vi "PWM Servo position FPGA.vi"() -> ()   [LabVIEW 2014]
doc: "This VI shows an example of how to implement a closed loop position move using the NI 9505. The position loop is implemented using PID. The output of the loop is used as the command for the current loop, which then sets the PWM duty cycle for the motor. This example assumes that an encoder is connected for position and velocity feedback. This example does not implement advanced motion features such as trajectory generation and splining."
uses:
  <vilib>/LabVIEW Targets/FPGA/cRIO/cRIO-9505/controls.llb/_nicrio_cRIO-9505_DriveStatus.ctl
  <vilib>/Platform/TimedLoop/XDataNode/timing_clust.ctl
  <vilib>/Platform/TimedLoop/XDataNode/nitl_modes.ctl
  <vilib>/Platform/TimedLoop/XDataNode/wakeup.ctl
  <vilib>/LabVIEW Targets/FPGA/cRIO/cRIO-9505/controls.llb/_nicrio_cRIO-9505_DriveDirection.ctl
  <vilib>/rvi/Emulation/niFpgaGetClockAttributes.vi
  <vilib>/rvi/Emulation/niFpgaSctlEmulationGetInTimedLoop.vi
  <vilib>/rvi/Emulation/niFpgaEmulationReportErrorSimple.vi
  <vilib>/rvi/eio/common/nirviEmuTemplateMethod_errors.vi
  <vilib>/rvi/eio/common/nirviEmuTemplatePropertyGet_noerrors.vi
  <vilib>/rvi/Emulation/niFpgaCriticalErrorInLSC.vi
  <vilib>/rvi/Emulation/niFpgaProcessEmulError.vi
  Instance           3 55Saved   Position Control (closed loop) - NI 9505 (FPGA) .vi
  Instance           4 55Saved   Position Control (closed loop) - NI 9505 (FPGA) .vi
  Instance           1 55Saved   Position Control (closed loop) - NI 9505 (FPGA) .vi
  Instance           2 55Saved   Position Control (closed loop) - NI 9505 (FPGA) .vi
  <vilib>/eio/EIOMethodNode/EIOMethodNode.xnode
  <vilib>/eio/EIOPropertyNode/EIOPropertyNode.xnode
  <vilib>/Platform/TimedLoop/XDataNode/XDataNode.xnode
  <vilib>/eio/EIONode/EIONode.xnode
  <vilib>/Platform/TimedLoop/XDataNode/XDNodeRunTimeDep.lvlib
  <vilib>/rvi/eio/common/nirviEmuTemplatePropertyGet_errors.vi
  <vilib>/rvi/eio/common/nirviEmuTemplatePropertySet_errors.vi
  <vilib>/rvi/eio/common/nirviEmuTemplatePropertySet_noerrors.vi
panel:
  out "Vsup Present":bool
  out "Drive Fault":bool
  out "Drive Status":T1=enum."Disabled"
  out "Temp Fault":bool
  in  "Enable\nDrive":bool
  in  "Disable\nDrive":bool
  in  "Reset Position":bool
  in  "Reset Position Value":i32
  out "Encoder Position":i32
  out "ticks/count":u32
  out "Index (Z) Position":i32
  out "counts (no reset)":i32
  in  "Position Loop  Rate (usec)":u16=250
  in  "Position PID Gains":T2={"Kp"=100, "Kd"=1000, "Ki"=0, "ILim"=1000, "Kv"=0, "Vff"=0, "Aff"=0, "Td"=2}
  in  "Position Error Limit":i16=32767
  out "Position Error Read":i16
  out "Position Error Status":bool
  in  "Position Setpoint":i32 caption="Setpoint"
  in  "Current PI Gains":T3={"Proportional Gain"=20, "Integral Gain"=10, "Derivative Gain"=0}
  in  "Current Limit":i16 caption="Setpoint"
  in  "Current Loop\nRate (usec)":u32=50
  in  "Trig AI":bool
  in  "Current Feedback":i16
  out "Current Loop Output":i16
  out "Current Command":i16
  # "VI Execution\nThis VI should be run with \"Position Control (closed loop) - NI 9505 (RT).vi\"."
  # "These parameters control the response of the position loop. Position Setpoint is the desired position to go to. Position Error Limit is the maximum allowed error the setpoint and actual position returned by the encoder loop."
  # "These parameters control the response\nof the current loop. The current limit is the \nmaximum current allowed."
  # "Kp: 3000\nKd: 2000\nKi: 1000\nILim: 1\n\nLoop rate: 50\nLimit: 100"
  # "Use the Reset Position control to reset the quadrature count to the value in Reset Position Value."
  # "These status controls/indicators are used to enable/disable the drive and read fault information."
  # "Drive Status"
  # "Encoder Parameters"
  # "Position Loop Parameters"
  # "Current Loop Parameters"
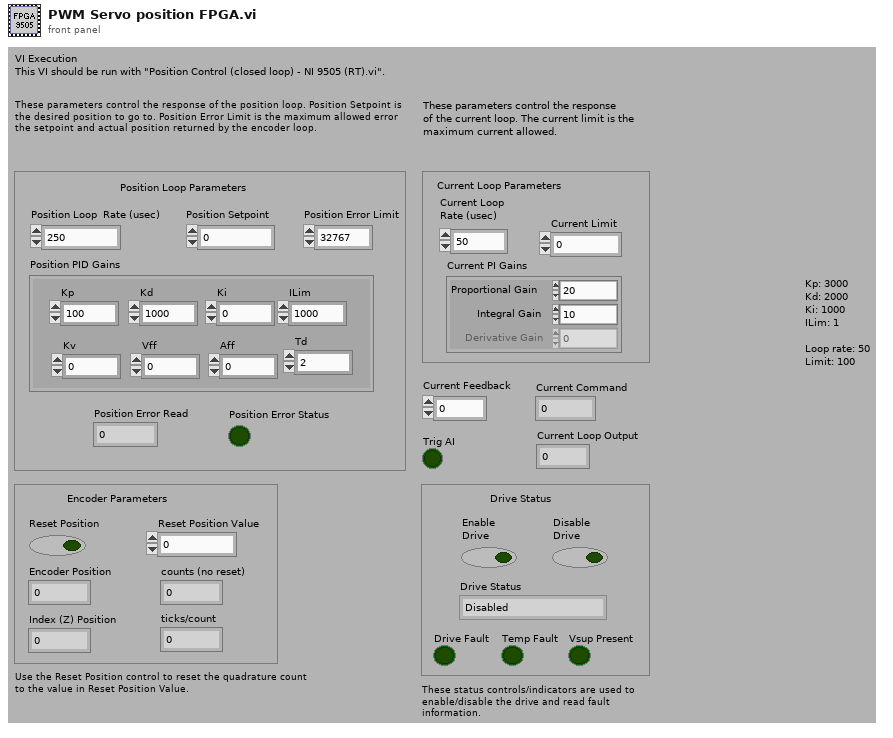
[diagram p1: front panel]
types:
  T1 = typedef "_nicrio_cRIO-9505_DriveStatus.ctl" = enum8{"Enabled", "Disabled", "Disabled by Drive Fault", "Disabled by Temp. Fault", "Disabled by E-Stop", "Unknown"}
  T2 = cluster{"Kp":i16, "Kd":i16, "Ki":i16, "ILim":i16, "Kv":i16, "Vff":i16, "Aff":i16, "Td":i16}
  T3 = cluster{"Proportional Gain":i16, "Integral Gain":i16, "Derivative Gain":i16}
  T4 = typedef "XDNodeRunTimeDep.lvlib/timing_clust.ctl" = cluster{"Expected End [f-1]":u64, "Actual End [f-1]":u64, "Finished Late? [f-1]":bool, "Expected End [i-1]":u64, "Actual End [i-1]":u64, "Finished Late? [i-1]":bool, "Expected Start [i]":u64, "Actual Start [i]":u64, "Expected Start [f]":u64, "Actual Start [f]":u64, "Source Name":string, "Structure Name":string, "Period":i64, "Deadline":i64, "Offset":i64, "Start":i64, "Priority":i32, "Timeout":i32, "Mode":T5, "Wakeup Reason":T6, "Error":errorcluster, "Source Type":string, "Secondary Source Type":string, "Global End Time":u64, "Global Start Time":u64, "Frame Duration":u64, "Iteration Duration":u64, "Assigned CPU":i32, "I/O Scan Engine Mode":u32}
  T5 = typedef "XDNodeRunTimeDep.lvlib/nitl_modes.ctl" = enum32{"No Change", "Process missed periods, maintain original phase", "Discard missed periods, maintain original phase", "Process missed periods, ignore original phase", "Discard missed periods, ignore original phase"}
  T6 = typedef "XDNodeRunTimeDep.lvlib/wakeup.ctl" = enum32{"Normal", "Aborted", "Asynchronous wakeup", "Timing source error", "Timed loop error", "Timeout"}
  T7 = typedef "_nicrio_cRIO-9505_DriveDirection.ctl" = enum8{"Clockwise", "Counterclockwise"}
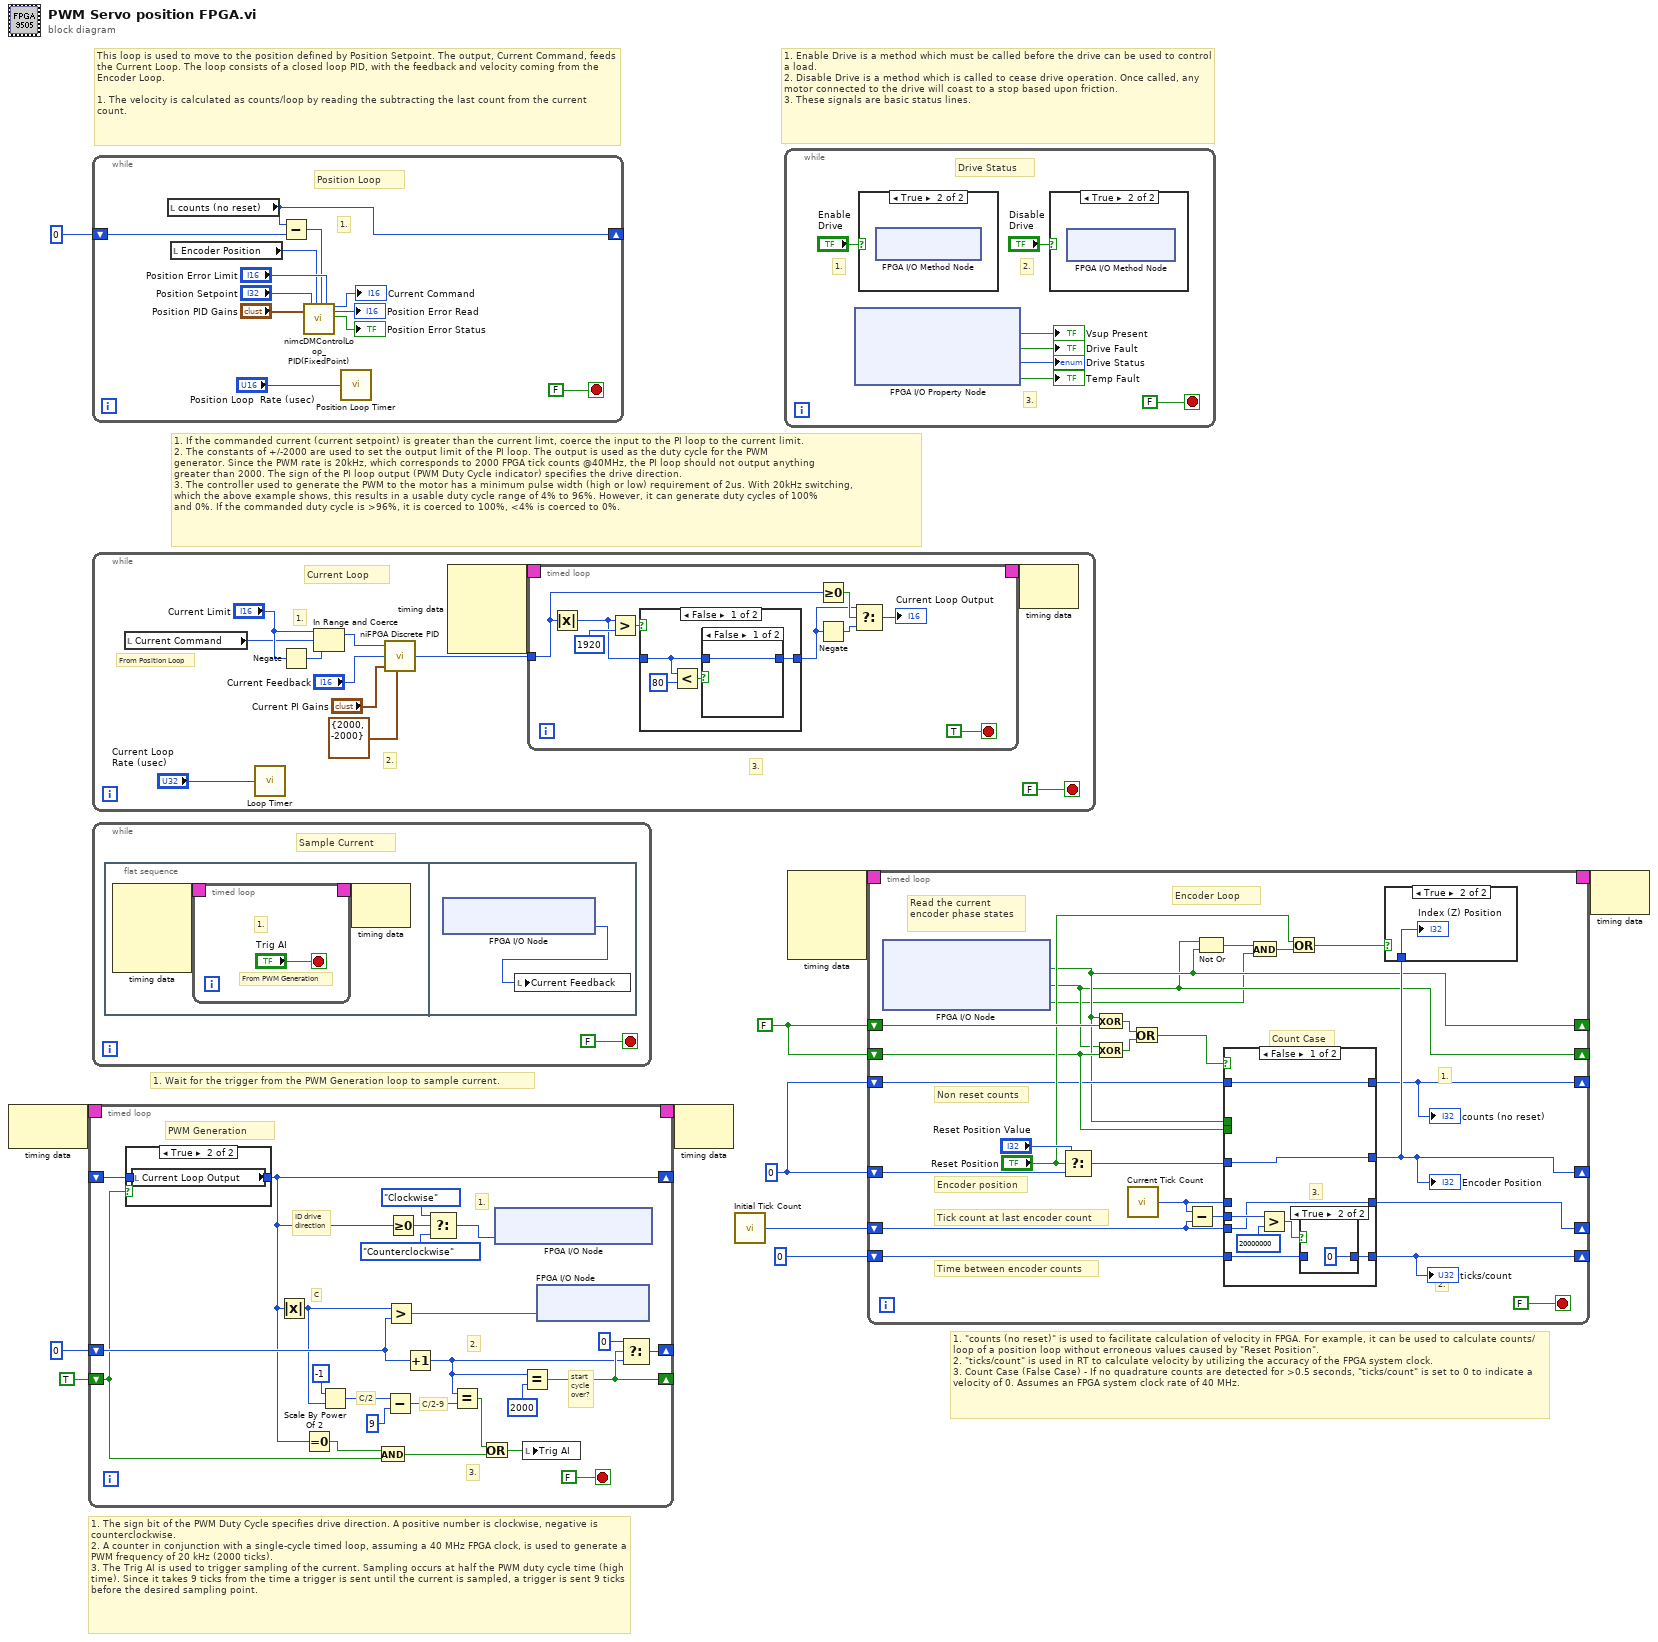
[diagram p0: block diagram]
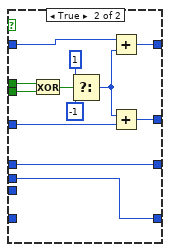
[diagram p4: hidden frame]
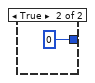
[diagram p6: hidden frame]
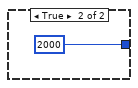
[diagram p7: hidden frame]
diagram:
  w2 = 0 ("Reset Position Value")
  w5 = FALSE ("Encoder Phase A")
  # "1. \"counts (no reset)\" is used to facilitate calculation of velocity in FPGA. For example, it can be used to calculate counts/loop of a position loop without erroneous values caused by \"Reset Position\". \n2. \"ticks/count\" is used in RT to calculate velocity by utilizing the accuracy of the FPGA system clock.\n3. Count Case (False Case) - If no quadrature counts are detected for >0.5 seconds, \"ticks/count\" is set to 0 to indicate a velocity of 0. Assumes an FPGA system clock rate of 40 MHz."
  # "1. Enable Drive is a method which must be called before the drive can be used to control a load.\n2. Disable Drive is a method which is called to cease drive operation. Once called, any motor connected to the drive will coast to a stop based upon friction.\n3. These signals are basic status lines."
  # "This loop is used to move to the position defined by Position Setpoint. The output, Current Command, feeds the Current Loop. The loop consists of a closed loop PID, with the feedback and velocity coming from the Encoder Loop.\n\n1. The velocity is calculated as counts/loop by reading the subtracting the last count from the current count."
  # "1. The sign bit of the PWM Duty Cycle specifies drive direction. A positive number is clockwise, negative is counterclockwise. \n2. A counter in conjunction with a single-cycle timed loop, assuming a 40 MHz FPGA clock, is used to generate a PWM frequency of 20 kHz (2000 ticks).\n3. The Trig AI is used to trigger sampling of the current. Sampling occurs at half the PWM duty cycle time (high time). Since it takes 9 ticks from the time a trigger is sent until the current is sampled, a trigger is sent 9 ticks before the desired sampling point."
  # "1. Wait for the trigger from the PWM Generation loop to sample current."
  # "1. If the commanded current (current setpoint) is greater than the current limt, coerce the input to the PI loop to the current limit.\n2. The constants of +/-2000 are used to set the output limit of the PI loop. The output is used as the duty cycle for the PWM\ngenerator. Since the PWM rate is 20kHz, which corresponds to 2000 FPGA tick counts @40MHz, the PI loop should not output anything\ngreater than 2000. The sign of the PI loop output (PWM Duty Cycle indicator) specifies the drive direction.\n3. The controller used to generate the PWM to the motor has a minimum pulse width (high or low) requirement of 2us. With 20kHz switching,\nwhich the above example shows, this results in a usable duty cycle range of 4% to 96%. However, it can generate duty cycles of 100%\nand 0%. If the commanded duty cycle is >96%, it is coerced to 100%, <4% is coerced to 0%."
  n1 = node-c288() -> (w11:T4)  [unwired: 1 out]
  n2 = timed-loop {
    timing: w11 -> [_]
    timing-out: [_] -> w10
    shift-right: [w32] -> _
    shift-left: i16 0 -> [w35]
    shift-right: [w31] -> _
    shift-left: TRUE -> [w28]
    shift-right: [w16] -> _
    shift-left: _ -> [w30]
    stop <- FALSE stop-if-true
    # "start \ncycle \nover?"
    # "C/2-9"
    # "C/2"
    # "C"
    # "ID drive\ndirection"
    # "3."
    # "2."
    # "1."
    # "PWM Generation"
    n3 = case shown="True" w28 {
      tunnel: [w36 w37] -> w16
      tunnel: w30 -> [w36 _]
      frame False {
      }
      frame True {
        n4 = local read "Current Loop Output"() -> (w37:i16)
      }
    }
    n5 = Absolute Value(x=w16) -> (abs(x)=w14:i16)
    n6 = Equal To 0?(x=w16) -> (x = 0?=w29:bool)
    n7 = Scale By Power Of 2(n=i8 -1, x=w14) -> (x*2^n=w18:i16)
    n8 = And(x=w29, y=w28) -> (x .and. y?=w25:bool)
    n9 = Subtract(x=w18, y=i8 9) -> (x-y=w17:i16)
    n10 = Greater?(x=w14, y=w35) -> (0:w12:bool)
    n11 = Greater Or Equal To 0?(x=w16) -> (x >= 0?=w24:bool)
    n12 = Increment(x=w35) -> (x+1=w27:i16)
    n13 = Select(t=_nicrio_cRIO-9505_DriveDirection."Clockwise" ("Drive Direction"), s=w24, f=_nicrio_cRIO-9505_DriveDirection."Counterclockwise" ("Drive Direction")) -> (s? t:f=w13:T7)
    n14 = Equal?(x=w27, y=w17) -> (x = y?=w26:bool)
    n15 = Or(x=w26, y=w25) -> (x .or. y?=w20:bool)
    n16 = xnode "FPGA I/O Node"("Mod7/Drive Direction"=w13) -> ()  [unwired: 1 in, 1 out]
    n17 = Equal?(x=w27, y=i16 2000) -> (x = y?=w31:bool)
    n18 = local write "Trig AI"(w20) -> ()
    n19 = xnode "FPGA I/O Node"("Mod7/Motor"=w12) -> ()  [unwired: 1 in, 1 out]
    n20 = Select(t=i16 0, s=w31, f=w27) -> (s? t:f=w32:i16)
  }
  n21 = while "Position Control Loop" {
    shift-right: [w43] -> _
    shift-left: 0 ("Encoder Position") -> [w45]
    stop <- FALSE stop-if-true
    # "1."
    # "Position Loop"
    n22 = local read "counts (no reset)"() -> (w43:i32)
    n23 = local read "Encoder Position"() -> (w40:i32)
    n24 = Subtract(x=w43, y=w45) -> (x-y=w44:i32)
    n25 = call "nimcDMControlLoop_PID(FixedPoint).vi"("PID Gains"="Position PID Gains", "Setpoint"="Position Setpoint", "Position Feedback"=w40, "Velocity Feedback"=w44, "Position Error Limit"="Position Error Limit") -> ("Output"=→"Current Command":i16, "Position Error Read"=→"Position Error Read":i16, "Position Error Status"=→"Position Error Status":bool)  [unwired: 2 in, 10 out]
    n26 = call "Position Loop Timer"("Count(uSec)"="Position Loop  Rate (usec)") -> ()  [unwired: 1 out]
  }
  n27 = while {
    stop <- FALSE stop-if-true
    # "From Position Loop"
    # "3."
    # "2."
    # "1."
    # "Current Loop"
    n28 = local read "Current Command"() -> (w52:i16)
    n29 = call "Loop Timer"("Count(uSec)"="Current Loop\nRate (usec)") -> ()  [unwired: 1 out]
    n30 = Negate(x="Current Limit") -> (-x=w56:i16)
    n31 = In Range and Coerce(upper limit="Current Limit", x=w52, lower limit=w56) -> (coerced(x)=w54:i16)  [unwired: 1 out]
    n32 = call <vilib>:"niFPGA Discrete PID.vi"("setpoint"=w54, "process variable"="Current Feedback", "PID gains (x 2^8)"="Current PI Gains", "output range"=cluster{"output high":i16, "output low":i16} {"output high"=2000, "output low"=-2000}) -> ("output"=w59:i16)  [unwired: 1 in, 4 out]
    n33 = node-c288() -> (w58:T4)  [unwired: 4 out]
    n34 = timed-loop {
      timing: w58 -> [_]
      timing-out: [_] -> w57
      tunnel: w59 -> [w66]
      stop <- TRUE stop-if-true
      n35 = Absolute Value(x=w66) -> (abs(x)=w67:i16)
      n36 = Greater?(x=w67, y=i16 1920 ("upper limit")) -> (0:w69:bool)
      n37 = case shown="False" w69 {
        tunnel: [w75 i16 2000 ("upper limit")] -> w68
        tunnel: w67 -> [w73 _]
        frame False {
          n38 = Less?(x=w73, y=i16 80 ("lower limit")) -> (x < y?=w74:bool)
          n39 = case shown="False" w74 {
            tunnel: [w77 i16 0 ("upper limit")] -> w75
            tunnel: w73 -> [w77 _]
            frame False {
            }
            frame True {
            }
          }
        }
        frame True {
        }
      }
      n40 = Greater Or Equal To 0?(x=w66) -> (x >= 0?=w72:bool)
      n41 = Negate(x=w68) -> (-x=w71:i16)
      n42 = Select(t=w68, s=w72, f=w71) -> (s? t:f=→"Current Loop Output":i16)
    }
    n43 = node-c288(w57) -> ()  [unwired: 1 out]
  }
  n44 = while {
    stop <- FALSE stop-if-true
    # "Sample Current"
    n45 = flat-sequence {
      frame #0 {
        n46 = node-c288() -> (w86:T4)  [unwired: 4 out]
        n47 = timed-loop {
          timing: w86 -> [_]
          timing-out: [_] -> w85
          stop <- "Trig AI" stop-if-true
          # "From PWM Generation"
          # "1."
        }
        n48 = node-c288(w85) -> ()  [unwired: 1 out]
      }
      frame #1 {
        n49 = xnode "FPGA I/O Node"() -> ("Mod7/Current Sense"=w92:i16)  [unwired: 1 in, 1 out]
        n50 = local write "Current Feedback"(w92) -> ()
      }
    }
  }
  n51 = node-c288(w10) -> ()  [unwired: 1 out]
  n52 = call "Initial Tick Count"() -> ("Tick Count(Ticks)"=w4:u32)
  n53 = while {
    stop <- FALSE stop-if-true
    # "Drive Status"
    # "3."
    # "2."
    # "1."
    n54 = xnode "FPGA I/O Property Node"() -> ("Vsup Present"=→"Vsup Present":bool, "Drive Fault"=→"Drive Fault":bool, "Drive Status"=→"Drive Status":T1, "Over Temperature Fault"=→"Temp Fault":bool)  [unwired: 1 in, 1 out]
    n55 = case shown="True" "Enable\nDrive" {
      frame False {
      }
      frame True {
        n56 = xnode "FPGA I/O Method Node"() -> ()  [unwired: 1 in, 1 out]
      }
    }
    n57 = case shown="True" "Disable\nDrive" {
      frame False {
      }
      frame True {
        n58 = xnode "FPGA I/O Method Node"() -> ()  [unwired: 1 in, 1 out]
      }
    }
  }
  n59 = node-c288() -> (w9:T4)  [unwired: 4 out]
  n60 = timed-loop {
    shift-right: [w102] -> _
    shift-left: w5 -> [w124]
    shift-right: [w101] -> _
    shift-left: w5 -> [w108]
    shift-right: [w110] -> _
    shift-left: w2 -> [w121]
    shift-right: [w117] -> _
    shift-left: w4 -> [w104]
    shift-right: [w116] -> _
    shift-left: u32 0 -> [w115]
    timing: w9 -> [_]
    timing-out: [_] -> w8
    shift-right: [w106] -> _
    shift-left: w2 -> [w107]
    stop <- FALSE stop-if-true
    # "Count Case"
    # "Encoder Loop"
    # "2."
    # "1."
    # "Read the current\nencoder phase states"
    # "Non reset counts"
    # "Encoder position"
    # "Time between encoder counts"
    # "Tick count at last encoder count"
    n61 = xnode "FPGA I/O Node"() -> ("Mod7/Encoder Phase A"=w102:bool, "Mod7/Encoder Phase B"=w101:bool, "Mod7/Encoder Index"=w100:bool)  [unwired: 3 in, 3 out]
    n62 = Select(t="Reset Position Value", s="Reset Position", f=w121) -> (s? t:f=w119:i32)
    n63 = Exclusive Or(1:w124, 2:w102) -> (0:w123:bool)
    n64 = Exclusive Or(1:w108, 2:w101) -> (0:w122:bool)
    n65 = call "Current Tick Count"() -> ("Tick Count(Ticks)"=w105:u32)
    n66 = Or(x=w123, y=w122) -> (x .or. y?=w120:bool)
    n67 = Subtract(x=w105, y=w104) -> (x-y=w103:u32)
    n68 = Not Or(1:w102, 2:w101) -> (0:w112:bool)
    n69 = case shown="False" w120 {
      tunnel: [w133 w141] -> w110
      tunnel: w119 -> [w133 w147]
      tunnel: w105 -> [_ w137]
      tunnel: [w128 w137] -> w117
      tunnel: w104 -> [w128 _]
      tunnel: [w126 w136] -> w116
      tunnel: w115 -> [w127 _]
      tunnel: w102 -> [_ w143]
      tunnel: w108 -> [_ w142]
      tunnel: [w132 w139] -> w106
      tunnel: w107 -> [w132 w138]
      tunnel: w103 -> [w129 w136]
      frame False {
        # "3."
        n70 = Greater?(x=w129, y=20000000 ("x")) -> (0:w130:bool)
        n71 = case shown="True" w130 {
          tunnel: [w134 u32 0] -> w126
          tunnel: w127 -> [w134 _]
          frame False {
          }
          frame True {
          }
        }
      }
      frame True {
        n72 = Exclusive Or(1:w142, 2:w143) -> (0:w144:bool)
        n73 = Select(t=1 ("16 bit"), s=w144, f=-1 ("16 bit")) -> (s? t:f=w140:i32)
        n74 = Add(x=w138, y=w140) -> (x+y=w139:i32)
        n75 = Add(x=w140, y=w147) -> (x+y=w141:i32)
      }
    }
    "Encoder Position" <- w110
    "ticks/count" <- w116
    "counts (no reset)" <- w106
    n76 = And(x=w112, y=w100) -> (x .and. y?=w113:bool)
    n77 = Or(x="Reset Position", y=w113) -> (x .or. y?=w111:bool)
    n78 = case shown="True" w111 {
      tunnel: w110 -> [_ w125]
      frame False {
      }
      frame True {
        "Index (Z) Position" <- w125
      }
    }
  }
  n79 = node-c288(w8) -> ()  [unwired: 1 out]
